vi "SaveFileToBMP(subVI).vi"(0 "WFGraph Refnum":refnum<vi>) -> ()   [LabVIEW 2026]
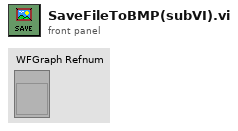
[diagram p1: front panel]
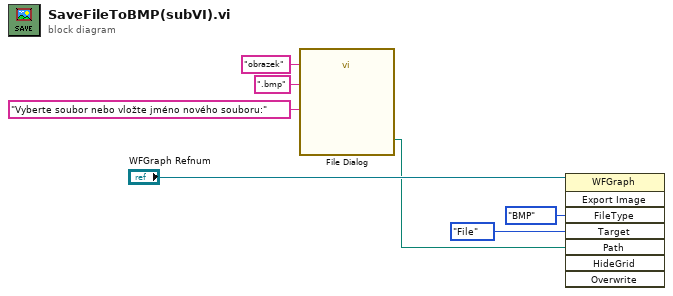
[diagram p0: block diagram]
diagram:
  n1 = call "File Dialog"("prompt"="Vyberte soubor nebo vložte jméno nového souboru:", "default name"="obrazek", "pattern (all files)"=".bmp") -> ("selected path"=w2:path)  [unwired: 9 in, 3 out]
  n2 = invoke class="WFGraph" method="Export Image"(reference="WFGraph Refnum", "FileType"=enum32{"BMP", "EPS", "EMF", "PICT"}."BMP" ("File Type"), "Target"=enum32{"File", "Clipboard"}."File", "Path"=w2) -> ()  [unwired: 4 in, 8 out]
